vi "GetIdentifier.vi"(8 "error in (no error)":errorcluster, 11 "DocumentClass in":refnum<class "Document.lvclass">) -> (0 "error out":errorcluster, 2 "Identifier":string, 3 "DocumentClass out":refnum<class "Document.lvclass">)   [LabVIEW 2021, in "ProligentXMLGenerator.lvlib" / "Document.lvclass"]
doc: "This document is uniquely identified by its Identifier.\n\nGUID Type."
uses:
  Document.lvclass
  Document.lvclass/Document.ctl
  Base/Guid/Guid.lvclass
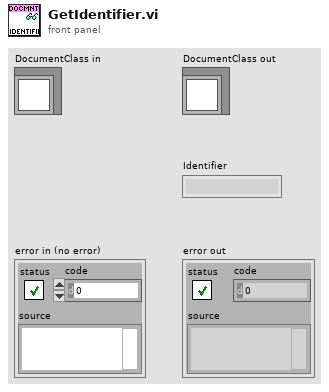
[diagram p1: front panel]
types:
  T1 = typedef "ProligentXMLGenerator.lvlib/Document.lvclass/Data.ctl" = cluster{"Name":string, "CustomData":refnum<class "CustomData.lvclass">, "Identifier":refnum<class "Guid.lvclass">, "NameType":refnum<class "NonEmptyString_255.lvclass">, "FileName":refnum<class "NonEmptyString_255.lvclass">, "Description":refnum<class "NonNullableString_600.lvclass">, "FilePath":path, "DestinationFolder":path}
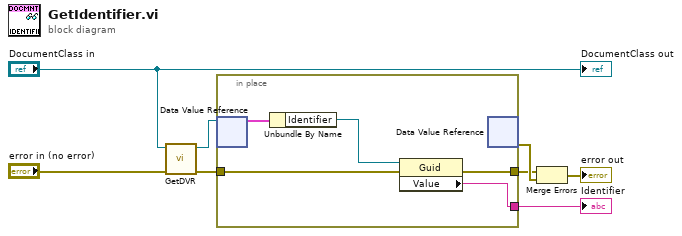
[diagram p0: block diagram]
diagram:
  n1 = call "GetDVR.vi"("error in"="error in (no error)", "Document in"="DocumentClass in") -> ("error out"=w5:errorcluster, "DVRReference"=w7:refnum<data-value>)  [unwired: 8 in]
  n2 = in-place "In Place Element Structure" {
    in-place-border: [w10] -> w6
    in-place-border: w5 -> [w11]
    in-place-border: [w9] -> w4
    n3 = in-place-dvr #1(w7) -> (w13:T1)  [unwired: 1 out]
    n4 = Unbundle By Name(w13) -> ("Identifier"=w12:refnum<class "Guid.lvclass">)
    n5 = property on="Property Node" class="Guid"(reference=w12, error in=w11) -> (error out=w9:errorcluster, "Value"=w10:string)  [unwired: 1 out]
    n6 = in-place-dvr #1() -> (w8:errorcluster)  [unwired: 1 in, 1 out]
  }
  "Identifier" <- w6
  n7 = Merge Errors(w4, w8) -> (→"error out":errorcluster)
  "DocumentClass out" <- "DocumentClass in"
